vi "autoDestroyFunction.vi"(11 "command in":string[](array[string])) -> ()   [LabVIEW 2012]
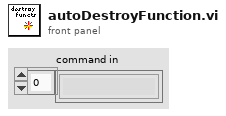
[diagram p1: front panel]
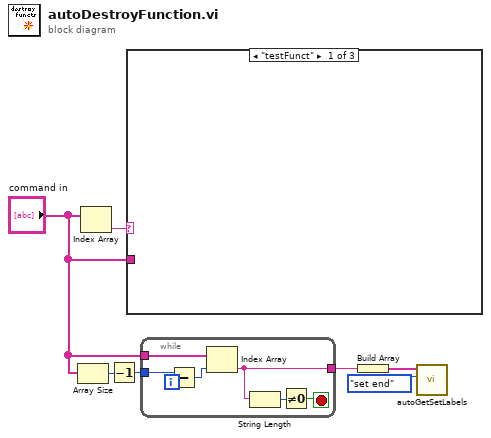
[diagram p0: block diagram]
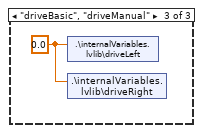
[diagram p3: hidden frame]
diagram:
  n1 = Array Size(array="command in") -> (size(s)=w6:i32)
  n2 = Index Array(array="command in") -> (element=w7:string)  [unwired: 1 in]
  n3 = Decrement(x=w6) -> (x-1=w5:i32)
  n4 = case shown="\"testFunct\"" w7 {
    tunnel: "command in" -> [_ _ _]
    frame "testFunct" {
    }
    frame Default {
    }
    frame "driveBasic", "driveManual" {
      w8 = 0.0 ("Output")
      n5 = shared-variable ".\\internalVariables.lvlib\\driveLeft"(w8) -> ()  [unwired: 1 in, 1 out]
      n6 = shared-variable ".\\internalVariables.lvlib\\driveRight"(w8) -> ()  [unwired: 1 in, 1 out]
    }
  }
  n7 = while {
    tunnel: "command in" -> [w13]
    tunnel: w5 -> [w14]
    tunnel: [w9] -> w2
    i -> [w15]
    stop <- w11 stop-if-true
    n8 = Subtract(x=w14, y=w15) -> (x-y=w12:i32)
    n9 = Index Array(array=w13, index=w12) -> (element=w9:string)
    n10 = String Length(string=w9) -> (length=w10:i32)
    n11 = Not Equal To 0?(x=w10) -> (x != 0?=w11:bool)
  }
  n12 = Build Array(w2) -> (w1:string[])
  n13 = call "autoGetSetLabels.vi"("option in"=enum16{"get", "set", "remove", "set end"}."set end", "label in"=w1) -> ()  [unwired: 9 in, 1 out]
